vi "Barcode 字數測試.vi"() -> ()   [LabVIEW 2019]
uses:
  <vilib>/regexp/Match Regular Expression.xnode
  LLB/Commonly VI/Main Glb.vi
  LLB/Commonly VI.lvlib
panel:
  out "substring":string
  out "after match":string
  out "before match":string
  out "result string":string
  in  "SN":string
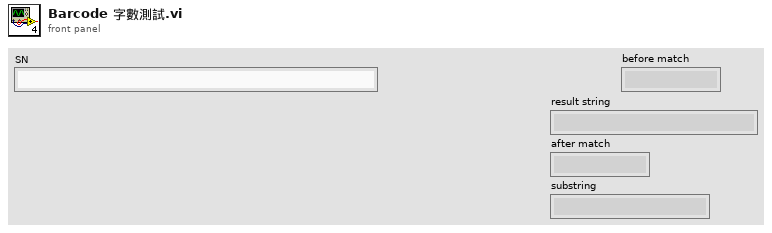
[diagram p1: front panel]
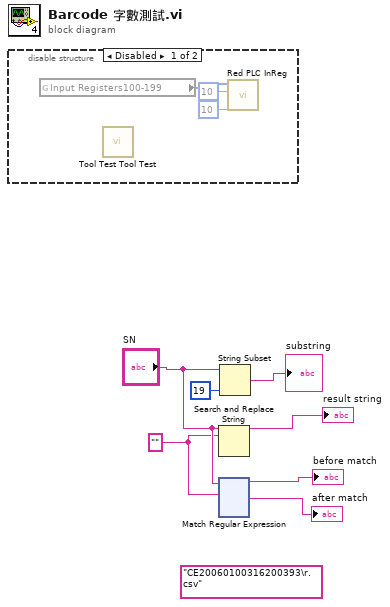
[diagram p0: block diagram]
diagram:
  w5 = "" ("search string")
  (unwired) "CE20060100316200393\r.csv"
  n1 = disable-structure shown="Disabled" {
    frame Disabled {
      n2 = global read "Main Glb.vi" "Input Registers100-199"() -> (w10:u16[])
      n3 = call "Tool Test Tool Test.vi"() -> ()  [unwired: 12 in]
      n4 = call "Red PLC InReg.vi"("length"=10, "index"=10, "Input Registers Arr"=w10) -> ()  [unwired: 8 in, 1 out]
    }
    frame Enabled {
    }
  }
  n5 = Search and Replace String(input string="SN", search string=w5) -> (result string=→"result string":string)  [unwired: 6 in, 3 out]
  n6 = xnode "Match Regular Expression"("input string"="SN", "regular expression"=w5) -> ("before match"=→"before match":string, "after match"=→"after match":string)  [unwired: 4 in, 3 out]
  n7 = String Subset(string="SN", length (rest)=19 ("length (rest)")) -> (substring=→"substring":string)  [unwired: 1 in]
